vi "DB write.vi"(2 "DB data":variant[][](array[variant]), 11 "DB write":T1) -> (6 "DB write":T1)   [LabVIEW 2023]
uses:
  <vilib>/addons/database/_DB Variant To Data/Database Variant To Data.xnode
panel:
  in  "Array":string[](array[string])=[" and MODELNAME='", " and PARTNO='", "and SR='", "and BARCODE='"]
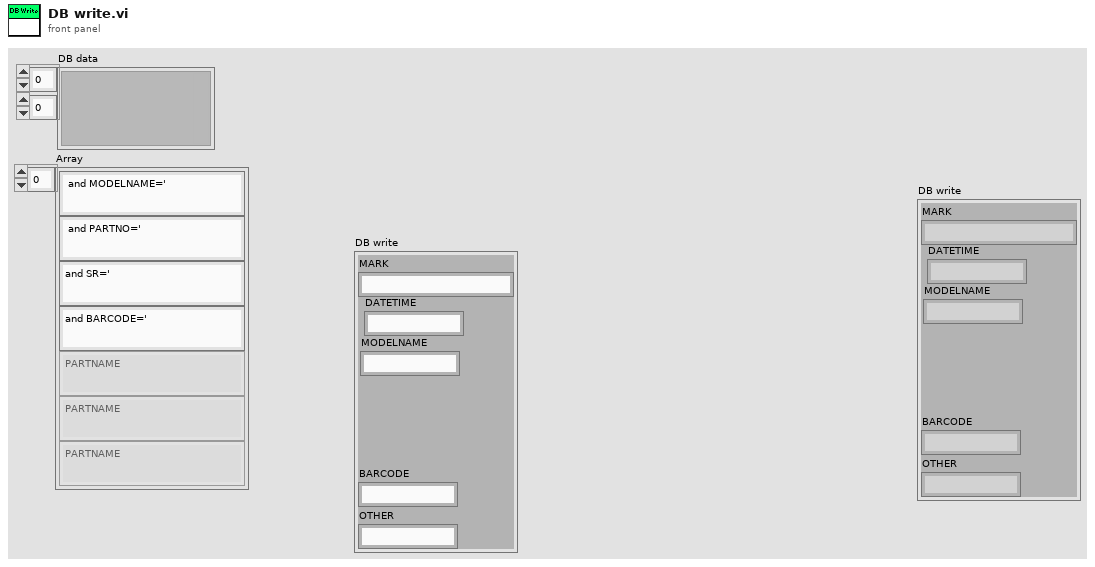
[diagram p1: front panel]
types:
  T1 = cluster{"DATETIME":string, "MODELNAME":string, "BARCODE":string, "MARK":string, "OTHER":string}
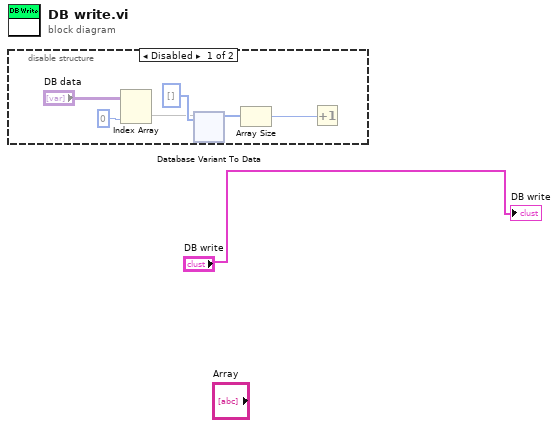
[diagram p0: block diagram]
diagram:
  n1 = disable-structure shown="Disabled" {
    frame Disabled {
      n2 = Index Array(array="DB data", index (col)=0 ("disabled index (col)")) -> (element=w4:variant[])  [unwired: 1 in]
      n3 = xnode "Database Variant To Data"("database variant"=w4, "type"=i32[] []) -> ("data"=w5:i32[])  [unwired: 1 in, 1 out]
      n4 = Array Size(array=w5) -> (size(s)=w7:i32)
      n5 = Increment(x=w7) -> ()  [unwired: 1 out]
    }
    frame Enabled {
    }
  }
  "DB write" <- "DB write"
